vi "0-Load Boat Icon.vi"() -> (0 "Array":u32[][](array[numeric]))   [LabVIEW 2011]
doc: "Loads the boat icon for use on the map. Also, replaces all the black pixels with transparent pixels."
panel:
  out "appended path":path
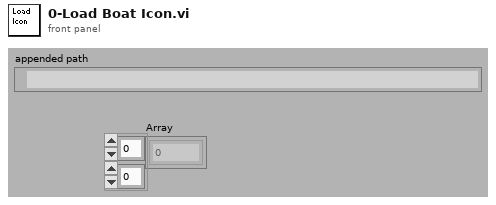
[diagram p1: front panel]
types:
  T1 = typedef "Image Type" = u32
  T2 = typedef "IMAQ Image.ctl" = refnum<image>
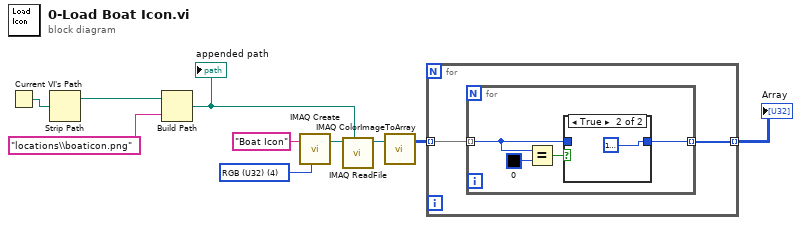
[diagram p0: block diagram]
diagram:
  w7 = T1 4 items=["Grayscale (U8)", "Grayscale (I16)", "Grayscale (SGL)", "Complex (CSG)", "RGB (U32)", "HSL (U32)", "RGB (U64)", "Grayscale (U16)"] ("Image Type")
  n1 = Current VI's Path() -> (path=w4:path)
  n2 = Strip Path(path=w4) -> (stripped path=w1:path)  [unwired: 1 out]
  n3 = Build Path(base path=w1, name or relative path="locations\\boaticon.png") -> (appended path=w2:path)
  "appended path" <- w2
  n4 = call "IMAQ Create"("Image Name"="Boat Icon", "Image Type"=w7) -> ("New Image"=w5:T2)  [unwired: 2 in, 2 out]
  n5 = call "IMAQ ReadFile"("File Path"=w2, "Image"=w5) -> ("Image Out"=w8:T2)  [unwired: 3 in, 6 out]
  n6 = call "IMAQ ColorImageToArray"("Image"=w8) -> ("Image Pixels (U32)"=w9:u32[][])  [unwired: 2 in, 3 out]
  n7 = for {
    tunnel: w9 -> [w12] mode=indexing
    tunnel: [w11] -> w10 mode=indexing
    n8 = for {
      tunnel: w12 -> [w13] mode=indexing
      tunnel: [w14] -> w11 mode=indexing
      n9 = Equal?(x=w13, y=u32 0) -> (x = y?=w16:bool)
      n10 = case shown="True" w16 {
        tunnel: [w17 u32 16777216] -> w14
        tunnel: w13 -> [w17 _]
        frame False {
        }
        frame True {
        }
      }
    }
  }
  "Array" <- w10
